vi "Configure Trigger (TV).vi"(0 "VISA resource name":refnum<visa-resource-name>, 1 "Signal Format (0: NTSC)":u16(ring) items=["NTSC", "PAL/SECAM"], 2 "TV Event (0: All Lines)":u16(ring) items=["All Lines", "Line Number", "Odd Field", "Even Field"], 5 "Trigger Source (1: Channel 1)":u16(ring)=1 items=["Channel 1"=1, "Channel 2"=2, "Channel 3"=3, "Channel 4"=4, "External"=5, "External 5"=6], 7 "TV Trigger Polarity (0: Positive)":u16(ring) items=["Positive", "Negative"], 9 "Trigger Modifier (0: Auto)":u16(ring) items=["Auto", "Normal", "Single"], 11 "error in (no error)":errorcluster, 12 "Trigger Level (0.0 V)":dbl, 13 "TV Line Number (1)":i32=1) -> (4 "VISA resource name out":refnum<visa-resource-name>, 15 "error out":errorcluster)   [LabVIEW 2010, in "Agilent DSO1000 Series.lvlib"]
doc: "Configures the TV trigger. You configure the TV trigger source, signal format, the event, and the signal polarity on which to trigger."
uses:
  <instrlib>/Agilent DSO1000 Series/Agilent DSO1000 Series.lvlib
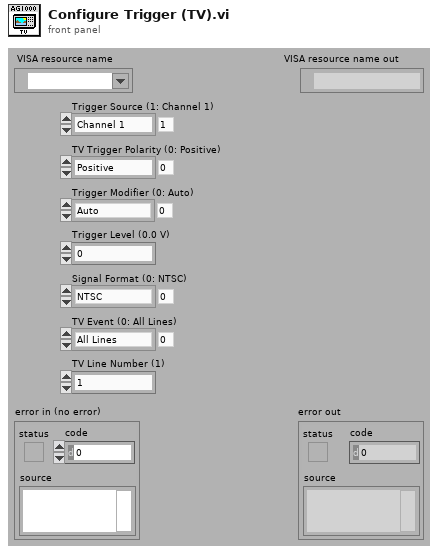
[diagram p1: front panel]
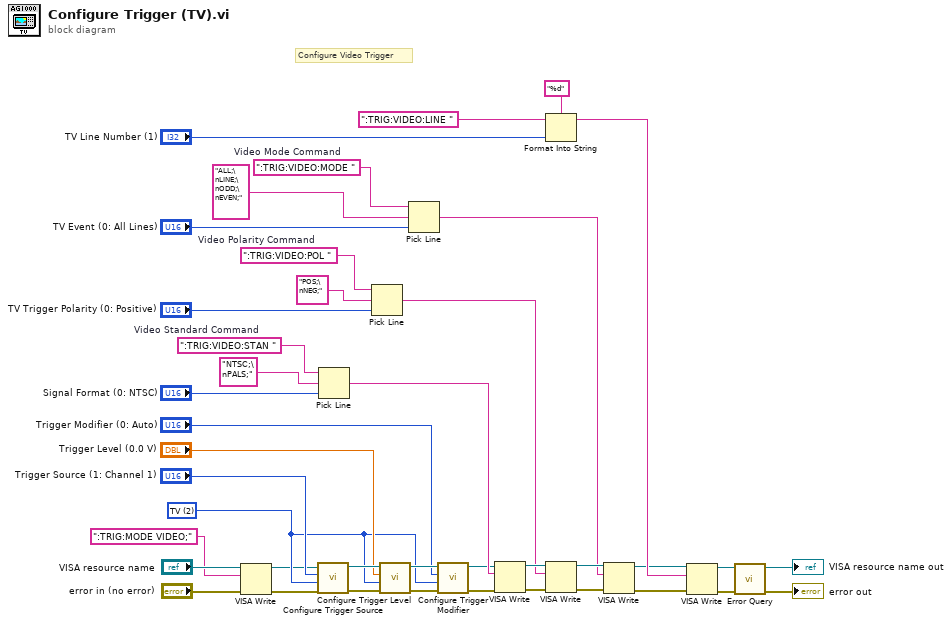
[diagram p0: block diagram]
diagram:
  w6 = u16 2 items=["Edge", "Pulse", "TV", "Pattern"] ("Trigger Type")
  w16 = ":TRIG:VIDEO:MODE "  # Video Mode Command
  w20 = ":TRIG:VIDEO:POL "  # Video Polarity Command
  w27 = ":TRIG:VIDEO:STAN "  # Video Standard Command
  # "Configure Video Trigger"
  n1 = VISA Write(VISA resource name="VISA resource name", write buffer=":TRIG:MODE VIDEO;", error in (no error)="error in (no error)") -> (VISA resource name out=w2:refnum<visa-resource-name>, error out=w4:errorcluster)  [unwired: 1 out]
  n2 = call <instrlib>:"Configure Trigger Source.vi"("error in (no error)"=w4, "Trigger Type"=w6, "Trigger Source (1: Channel 1)"="Trigger Source (1: Channel 1)", "VISA resource name"=w2) -> ("error out"=w35:errorcluster, "VISA resource name out"=w34:refnum<visa-resource-name>)  [unwired: 6 in]
  n3 = Pick Line(string ("")=w27, multi-line string="NTSC;\nPALS;", line index="Signal Format (0: NTSC)") -> (output string=w26:string)
  n4 = Pick Line(string ("")=w20, multi-line string="POS;\nNEG;", line index="TV Trigger Polarity (0: Positive)") -> (output string=w19:string)
  n5 = call <instrlib>:"Configure Trigger Level.vi"("error in (no error)"=w35, "Trigger Type"=w6, "Trigger Level (0.0 V)"="Trigger Level (0.0 V)", "VISA resource name"=w34) -> ("error out"=w32:errorcluster, "VISA resource name out"=w31:refnum<visa-resource-name>)  [unwired: 6 in]
  n6 = Pick Line(string ("")=w16, multi-line string="ALL;\nLINE;\nODD;\nEVEN;", line index="TV Event (0: All Lines)") -> (output string=w13:string)
  n7 = call <instrlib>:"Configure Trigger Modifier.vi"("error in (no error)"=w32, "Trigger Type"=w6, "Trigger Modifier (0: Auto)"="Trigger Modifier (0: Auto)", "VISA resource name"=w31) -> ("error out"=w24:errorcluster, "VISA resource name out"=w25:refnum<visa-resource-name>)  [unwired: 6 in]
  n8 = VISA Write(VISA resource name=w25, write buffer=w26, error in (no error)=w24) -> (VISA resource name out=w22:refnum<visa-resource-name>, error out=w23:errorcluster)  [unwired: 1 out]
  n9 = Format Into String(format string="%d", initial string=":TRIG:VIDEO:LINE ", "TV Line Number (1)") -> (resulting string=w9:string)  [unwired: 1 in, 1 out]
  n10 = VISA Write(VISA resource name=w22, write buffer=w19, error in (no error)=w23) -> (VISA resource name out=w14:refnum<visa-resource-name>, error out=w15:errorcluster)  [unwired: 1 out]
  n11 = VISA Write(VISA resource name=w14, write buffer=w13, error in (no error)=w15) -> (VISA resource name out=w8:refnum<visa-resource-name>, error out=w7:errorcluster)  [unwired: 1 out]
  n12 = VISA Write(VISA resource name=w8, write buffer=w9, error in (no error)=w7) -> (VISA resource name out=w39:refnum<visa-resource-name>, error out=w38:errorcluster)  [unwired: 1 out]
  n13 = call <instrlib>:"Error Query.vi"("error in (no error)"=w38, "VISA resource name"=w39) -> ("error out"=→"error out":errorcluster, "VISA resource name out"=→"VISA resource name out":refnum<visa-resource-name>)  [unwired: 6 in, 2 out]
